vi "Plot.vi"(8 "error in (no error)":errorcluster caption="에러 입력(에러 없음)", 9 "Histogram parameter":T1={"IEI Histo"={"Number of bin "=500.0, "Max."=10.0, "Min."=0.0}, "Freq Histo"={"Number of bin"=500.0, "Max."=60.0, "Min."=10.0}}, 11 "Data Stack IN":refnum<class "Retrieved Data.lvclass">[](array[class])) -> (0 "error out":errorcluster caption="에러 출력", 1 "Amplitude":cluster{"X Values":dbl[], dbl[]}[](graph), 2 "Interevent interval":cluster{"X Values":dbl[], dbl[]}[](graph), 3 "Data Stack OUT":refnum<class "Retrieved Data.lvclass">[](array[class]))   [LabVIEW 2017, in "Retrieved Data.lvclass"]
uses:
  Retrieved Data.lvclass
  Retrieved Data.lvclass/Retrieved Data.ctl
  <vilib>/Analysis/NI_AALPro.lvlib
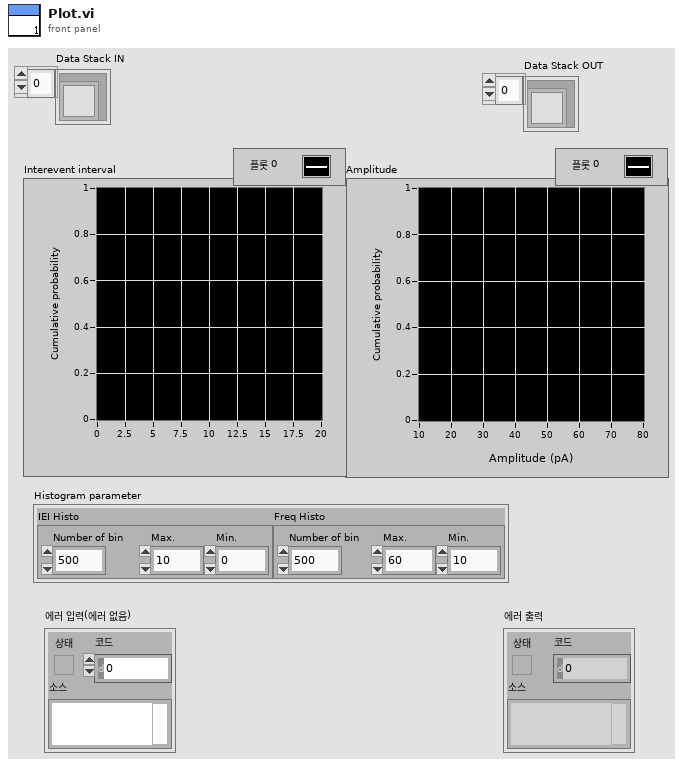
[diagram p1: front panel]
types:
  T1 = cluster{"IEI Histo":cluster{"Number of bin ":dbl, "Max.":dbl, "Min.":dbl}, "Freq Histo":cluster{"Number of bin":dbl, "Max.":dbl, "Min.":dbl}}
  T2 = cluster{"X Values":dbl[], "Histogram: h(x)":i32[]}
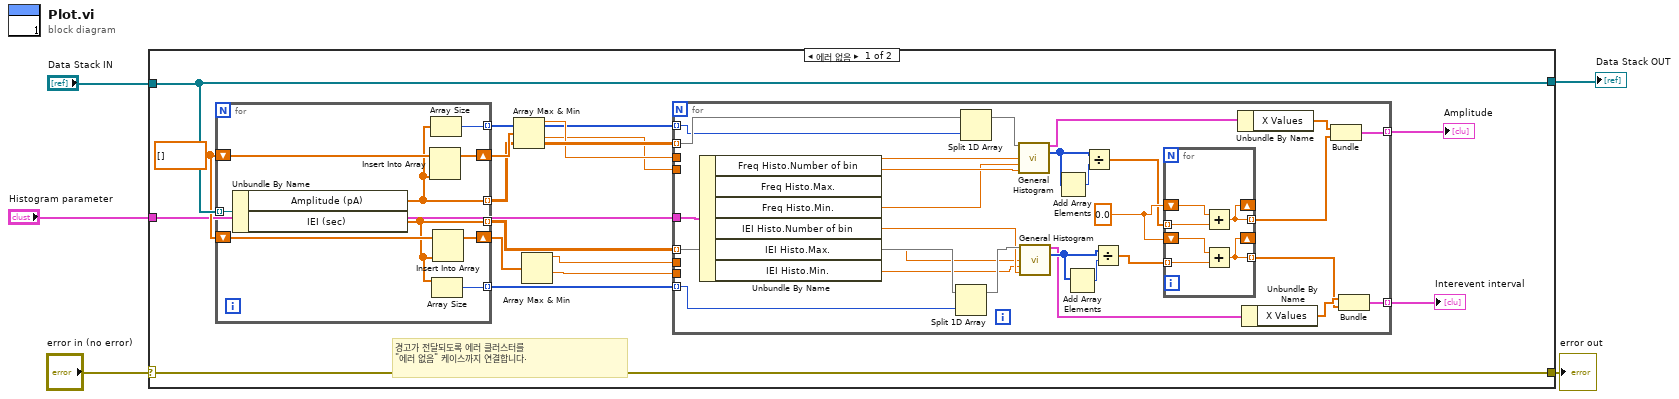
[diagram p0: block diagram]
diagram:
  n1 = case shown="에러 없음" "error in (no error)" {
    selector: "error in (no error)" -> [w21 w66]
    tunnel: [w21 w66] -> w4
    tunnel: [w20 w65] -> w2
    tunnel: "Data Stack IN" -> [w20 w65]
    tunnel: "Histogram parameter" -> [w6 _]
    frame No Error {
      w19 = dbl[] []
      # "경고가 전달되도록 에러 클러스터를\n\"에러 없음\" 케이스까지 연결합니다."
      n2 = for {
        tunnel: w20 -> [w64] mode=indexing
        tunnel: [w59] -> w16 mode=indexing
        tunnel: [w57] -> w15 mode=indexing
        shift-right: [w63] -> w18
        shift-left: w19 -> [w62]
        shift-right: [w61] -> w17
        shift-left: w19 -> [w60]
        tunnel: [w58] -> w8 mode=indexing
        tunnel: [w56] -> w7 mode=indexing
        n3 = Unbundle By Name(w64) -> ("Amplitude (pA)"=w59:dbl[], "IEI (sec)"=w57:dbl[])
        n4 = Insert Into Array(array=w62, new element=w59) -> (w63:dbl[])  [unwired: 1 in]
        n5 = Array Size(array=w59) -> (size(s)=w58:i32)
        n6 = Array Size(array=w57) -> (size(s)=w56:i32)
        n7 = Insert Into Array(array=w60, new element=w57) -> (w61:dbl[])  [unwired: 1 in]
      }
      n8 = Array Max & Min(array=w18) -> (max value=w14:dbl, min value=w13:dbl)  [unwired: 2 out]
      n9 = Array Max & Min(array=w17) -> (max value=w12:dbl, min value=w11:dbl)  [unwired: 2 out]
      n10 = for {
        tunnel: w16 -> [w34] mode=indexing
        tunnel: w15 -> [w32] mode=indexing
        tunnel: w14 -> [_]
        tunnel: w13 -> [_]
        tunnel: w12 -> [_]
        tunnel: w11 -> [_]
        tunnel: [w36] -> w10 mode=indexing
        tunnel: [w35] -> w9 mode=indexing
        tunnel: w8 -> [w30] mode=indexing
        tunnel: w7 -> [w29] mode=indexing
        tunnel: w6 -> [w28]
        w45 = 0.0
        n11 = Unbundle By Name(w28) -> ("Freq Histo.Number of bin"=w27:dbl, "Freq Histo.Max."=w24:dbl, "Freq Histo.Min."=w25:dbl, "IEI Histo.Number of bin"=w26:dbl, "IEI Histo.Max."=w22:dbl, "IEI Histo.Min."=w23:dbl)
        n12 = Split 1D Array(array=w32, index=w29) -> (first subarray=w31:dbl[])  [unwired: 1 out]
        n13 = Split 1D Array(array=w34, index=w30) -> (first subarray=w33:dbl[])  [unwired: 1 out]
        n14 = call <vilib>:"General Histogram.vi"("X"=w33, "max"=w24, "min"=w25, "# bins"=w27) -> ("Histogram Graph"=w42:T2, "Histogram"=w49:i32[])  [unwired: 7 in, 3 out]
        n15 = call <vilib>:"General Histogram.vi"("X"=w31, "max"=w22, "min"=w23, "# bins"=w26) -> ("Histogram Graph"=w41:T2, "Histogram"=w47:i32[])  [unwired: 7 in, 3 out]
        n16 = Add Array Elements(numeric array=w49) -> (sum=w48:i32)
        n17 = Add Array Elements(numeric array=w47) -> (sum=w46:i32)
        n18 = Divide(x=w49, y=w48) -> (x/y=w43:dbl[])
        n19 = Divide(x=w47, y=w46) -> (x/y=w44:dbl[])
        n20 = for {
          tunnel: w43 -> [w54] mode=indexing
          shift-right: [w53] -> _
          shift-left: w45 -> [w55]
          tunnel: [w53] -> w39 mode=indexing
          tunnel: w44 -> [w51] mode=indexing
          shift-right: [w50] -> _
          shift-left: w45 -> [w52]
          tunnel: [w50] -> w37 mode=indexing
          n21 = Add(x=w55, y=w54) -> (x+y=w53:dbl)
          n22 = Add(x=w52, y=w51) -> (x+y=w50:dbl)
        }
        n23 = Unbundle By Name(w42) -> ("X Values"=w40:dbl[])
        n24 = Unbundle By Name(w41) -> ("X Values"=w38:dbl[])
        n25 = Bundle("X Values"=w40, w39) -> (w36:cluster{"X Values":dbl[], dbl[]})  [unwired: 1 in]
        n26 = Bundle("X Values"=w38, w37) -> (w35:cluster{"X Values":dbl[], dbl[]})  [unwired: 1 in]
      }
      "Amplitude" <- w10
      "Interevent interval" <- w9
    }
    frame Error {
    }
  }
  "error out" <- w4
  "Data Stack OUT" <- w2
